vi "loadDBCReadSingal.vi"() -> ()   [LabVIEW 2016]
uses:
  CAN_Info.ctl
  CAN_BaudInfo.ctl
  CAN_FrameInfo.ctl
  TCANProperty.ctl
  SendMsgInfo.ctl
  D:/Program Files (x86)/TOSUN/TSMaster/bin/Data/SDK/lib/x86/TSMaster.dll
panel:
  in  "AAppChannel":i32(ring) items=["CHN1", "CHN2", "CHN3", "CHN4", "CHN5", "CHN6", "CHN7", "CHN8", "CHN9", "CHN10", "CHN11", "CHN12", "CHN13", "CHN14", "CHN15", "CHN16", "CHN17", "CHN18", "CHN19", "CHN20", "CHN21", "CHN22", "CHN23", "CHN24", "CHN25", "CHN26", "CHN27", "CHN28", "CHN29", "CHN30", "CHN31", "CHN32"]
  out "数值 2":u32
  in  "发送数据帧信息":T1={"AID"=1234, "AIsExt"=enum."STD", "AIsRemote"=enum."Data", "ADLC"=5, "ADataArray"=[0, 0, 10, 96, 8, 8]} {"ADLC" max=64; "AID" max=536870911}
  out "out AId":u32
  out "tsdb_load_can_db":i32
  out "tsdb_get_signal_value_can":i32
  in  "停止":bool
  out "错误输出":errorcluster
  out "数值":u32
  in  "配置波特率":T2={"ABaudrateKbps"=500.0, "AListenOnly"=enum."Normal", "Int120Ohm"=enum."Enable", "EnableChannel"=enum."Enable", "AAppChannel"=0, "硬件类型"=3, "AHwChannel"=0} {"AHwChannel" items=["CHN1", "CHN2", "CHN3", "CHN4", "CHN5", "CHN6", "CHN7", "CHN8", "CHN9", "CHN10", "CHN11", "CHN12", "CHN13", "CHN14", "CHN15", "CHN16", "CHN17", "CHN18", "CHN19", "CHN20", "CHN21", "CHN22", "CHN23", "CHN24", "CHN25", "CHN26", "CHN27", "CHN28", "CHN29", "CHN30", "CHN31", "CHN32", "CHN82"]; "硬件类型" items=["BUS_UNKNOWN_TYPE", "TS_TCP_DEVICE", "XL_USB_DEVICE", "TS_USB_DEVICE", "PEAK_USB_DEVICE", "KVASER_USB_DEVICE", "ZLG_USB_DEVICE", "ICS_USB_DEVICE", "TS_TC1005_DEVICE"]; "AAppChannel" items=["CHN1", "CHN2", "CHN3", "CHN4", "CHN5", "CHN6", "CHN7", "CHN8", "CHN9", "CHN10", "CHN11", "CHN12", "CHN13", "CHN14", "CHN15", "CHN16", "CHN17", "CHN18", "CHN19", "CHN20", "CHN21", "CHN22", "CHN23", "CHN24", "CHN25", "CHN26", "CHN27", "CHN28", "CHN29", "CHN30", "CHN31", "CHN32"]}
  out "ConnectSeccessfully":bool
  in  "CAN_CardProperties":T3={"应用程序名"="APP", "CAN使用通道数"=1, "LIN使用通道数"=0} {"LIN使用通道数" max=5; "CAN使用通道数" min=1 max=1 step=1}
  in  "ASupportedChannelsBased0":string="0"
  in  "路径":path=path "D:/安洁资料/B2-EP33L/201017-hd2-EP33L_EP1_WLC-V01.dbc"
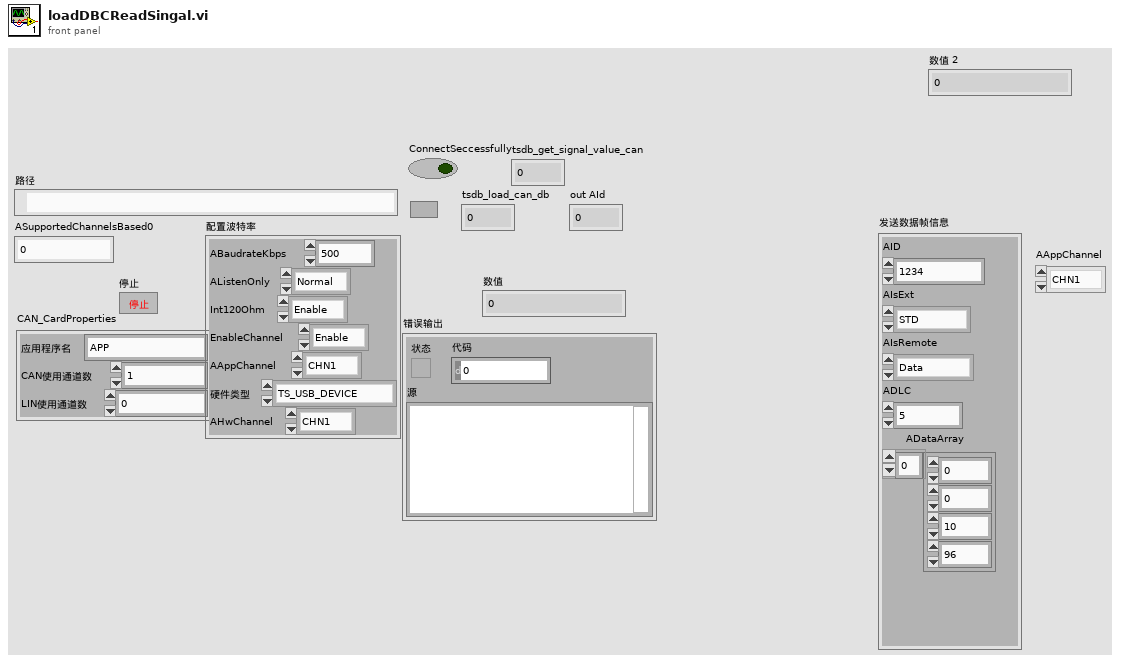
[diagram p1: front panel]
types:
  T1 = typedef "CAN_FrameInfo.ctl" = cluster{"AID":u32, "AIsExt":enum16{"STD", "EXT"}, "AIsRemote":enum16{"Data", "Remote"}, "ADLC":u8, "ADataArray":u8[]}
  T2 = typedef "CAN_BaudInfo.ctl" = cluster{"ABaudrateKbps":sgl, "AListenOnly":enum16{"Normal", "ListenOnly"}, "Int120Ohm":enum16{"Disable", "Enable"}, "EnableChannel":enum16{"Disable", "Enable"}, "AAppChannel":i32, "硬件类型":i32, "AHwChannel":i32}
  T3 = typedef "CAN_Info.ctl" = cluster{"应用程序名":string, "CAN使用通道数":u8, "LIN使用通道数":u8}
  T4 = typedef "SendMsgInfo.ctl" = cluster{"FIdxChn":u8, "FProperties":u8, "FDLC":u8, "FReserved":u8, "FIdentifier":i32, "FTimeUS":u64, "Data0":u8, "Data1":u8, "Data2":u8, "Data3":u8, "Data4":u8, "Data5":u8, "Data6":u8, "Data7":u8}
  T5 = typedef "TCANProperty.ctl" = cluster{"istx":bool, "remoteframe":bool, "extframe":bool, "tbd1":bool, "tbd2":bool, "tbd3":bool, "tbd4":bool, "iserrorframe":bool}
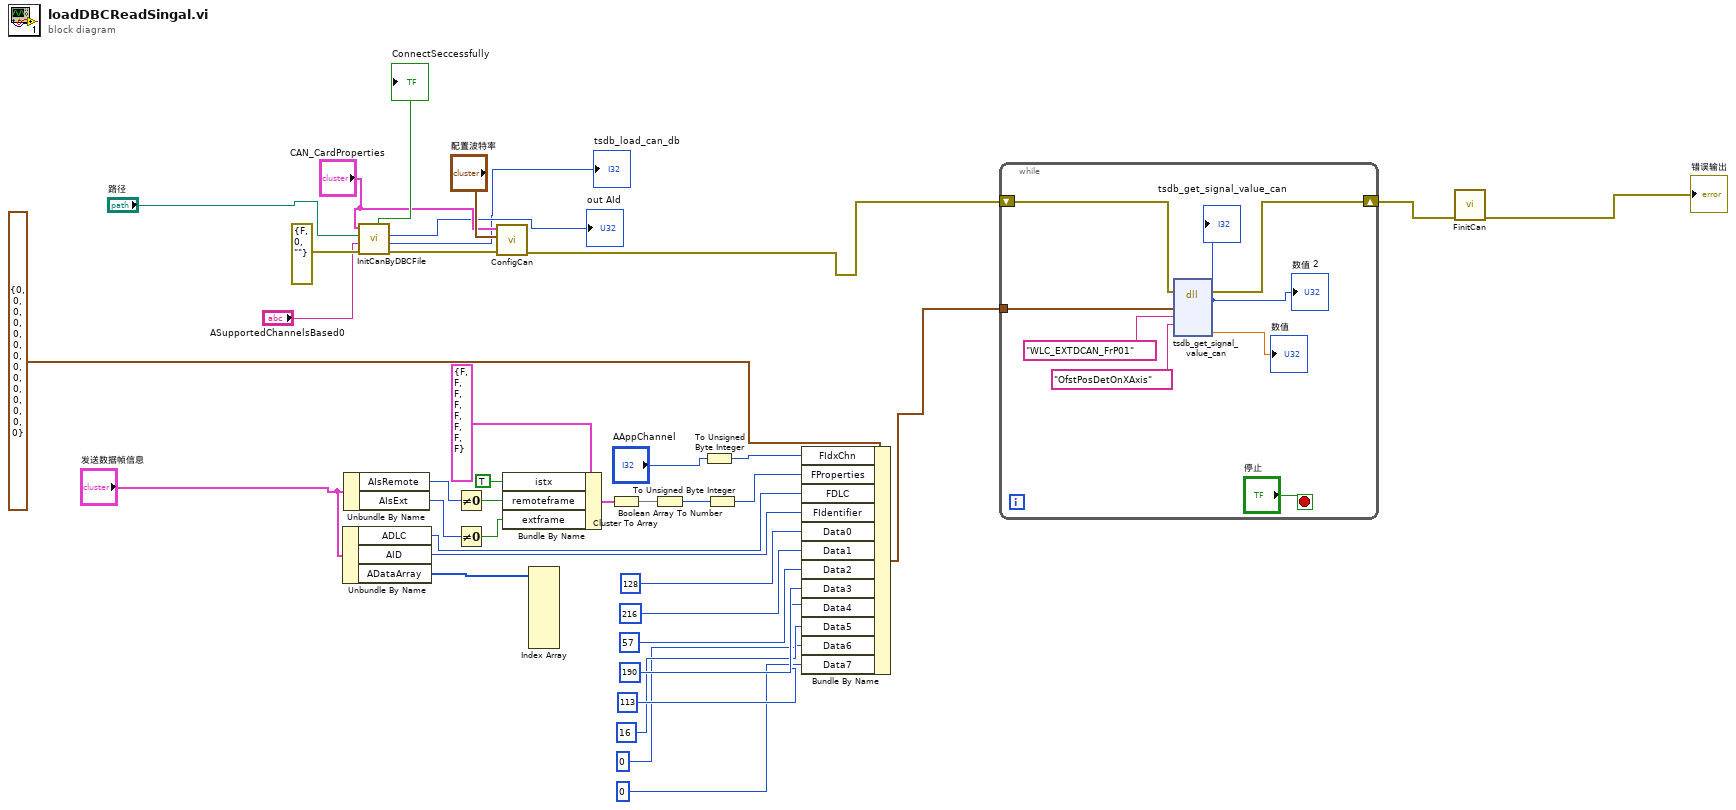
[diagram p0: block diagram]
diagram:
  n1 = Unbundle By Name("发送数据帧信息") -> ("ADLC"=w13:u8, "AID"=w12:u32, "ADataArray"=w11:u8[])
  n2 = Unbundle By Name("发送数据帧信息") -> ("AIsRemote"=w20:enum16{"Data", "Remote"}, "AIsExt"=w18:enum16{"STD", "EXT"})
  n3 = call "InitCanByDBCFile.vi"("错误输入"=errorcluster {"status"=FALSE, "code"=0, "source"=""}, "ASupportedChannelsBased0"="ASupportedChannelsBased0", "路径"="路径", "CAN_CardProperties"="CAN_CardProperties") -> ("错误输出"=w34:errorcluster, "tsdb_load_can_db"=→"tsdb_load_can_db":i32, "out AId"=→"out AId":u32, "ConnectSeccessfully"=→"ConnectSeccessfully":bool)  [unwired: 3 in, 1 out]
  n4 = Not Equal To 0?(x=w20) -> (x != 0?=w21:bool)
  n5 = Not Equal To 0?(x=w18) -> (x != 0?=w19:bool)
  n6 = call "ConfigCan.vi"("错误输入（无错误）"=w34, "配置波特率"="配置波特率", "CAN_CardProperties"="CAN_CardProperties") -> ("错误输出"=w27:errorcluster)  [unwired: 7 in, 1 out]
  n7 = Bundle By Name(cluster=T5 {"istx"=FALSE, "remoteframe"=FALSE, "extframe"=FALSE, "tbd1"=FALSE, "tbd2"=FALSE, "tbd3"=FALSE, "tbd4"=FALSE, "iserrorframe"=FALSE} ("TCANProperty"), "istx"=TRUE, "remoteframe"=w21, "extframe"=w19) -> (w17:T5)
  n8 = Index Array(array=w11) -> ()  [unwired: 8 in, 8 out]
  n9 = Cluster To Array(cluster=w17) -> (array=w16:bool[])
  n10 = Boolean Array To Number(Boolean array=w16) -> (number=w15:u32)
  n11 = To Unsigned Byte Integer(number="AAppChannel") -> (unsigned 8bit integer=w24:u8)
  n12 = To Unsigned Byte Integer(number=w15) -> (unsigned 8bit integer=w14:u8)
  n13 = Bundle By Name(cluster=T4 {"FIdxChn"=0, "FProperties"=0, "FDLC"=0, "FReserved"=0, "FIdentifier"=0, "FTimeUS"=0, "Data0"=0, "Data1"=0, "Data2"=0, "Data3"=0, "Data4"=0, "Data5"=0, "Data6"=0, "Data7"=0} ("SendMsgInfo"), "FIdxChn"=w24, "FProperties"=w14, "FDLC"=w13, "FIdentifier"=w12, "Data0"=u8 128 ("Data7"), "Data1"=u8 216 ("Data7"), "Data2"=u8 57 ("Data7"), "Data3"=u8 190 ("Data7"), "Data4"=u8 113 ("Data7"), "Data5"=u8 16 ("Data7"), "Data6"=u8 0 ("Data7"), "Data7"=u8 0) -> (w9:T4)
  n14 = while {
    shift-right: [w42] -> w36
    shift-left: w27 -> [w43]
    tunnel: w9 -> [w40]
    stop <- "停止" stop-if-true
    n15 = dll-call lib="D:/Program Files (x86)/TOSUN/TSMaster/bin/Data/SDK/lib/x86/TSMaster.dll" fn="tsdb_get_signal_value_can"(error in=w43, "ACAN"=w40, "AMsgName"="WLC_EXTDCAN_FrP01", "ASgnName"="OfstPosDetOnXAxis" ("AMsgName")) -> (error out=w42:errorcluster, "tsdb_get_signal_value_can"=→"tsdb_get_signal_value_can" →"数值 2":i32, "AValue"=→"数值":dbl)  [unwired: 6 in, 1 out]
  }
  n16 = call "FinitCan.vi"("错误输入（无错误）"=w36) -> ("错误输出"=→"错误输出":errorcluster)  [unwired: 10 in]
